vi "Filter(SubVI).vi"(0 "Horní mezní frekvence":dbl, 1 "Vstupní signál":waveform(dbl)[](array[waveform]), 2 "Druh filtru":T1, 3 "Dolní mezní frekvence":dbl, 4 "Vstup z registru":dbl[](array[numeric]), 5 "Typ filtru":bool) -> (6 "Signál":waveform(dbl)[](array[waveform]), 7 "Spektrum":cluster{"f0":dbl, "df":dbl, "magnitude":dbl[]}[](array[cluster]), 8 "Výstup filtrovaného signálu":dbl[](array[numeric]))   [LabVIEW 2025]
doc: "Celkem obsahuje 6 vstupů:\n 1. Vstupní signál pro filtraci\n 2. Horní mezní frekvenci filtru\n 3. Dolní mezní frekvenci filtru (jedinou mezní frekvenci pro filtry DP a HP)\n 4. Přepínač pro typ filtru\n 5. Výběr druhu filtru (HP, DP, PP, PZ)\n 6. Vstup pro kontrolu signálu\nObsahuje 3 výstupy:\n 1. Výstupní vyfiltrovaný signál + původní nefiltrovaný signál\n 2. Spektra obou signálů\n 3. Výstup filtrovaného signálu pro kontrolu\n\nV závislosti na pozici boolean tlačítka se využívá buď FIR filtr, pokud je tlačítko ve stavu OFF, nebo IIR filtr, pokud je tlačítko ve stavu ON."
uses:
  <vilib>/Analysis/NI_AALBase.lvlib
  <vilib>/measure/NI_MAPro.lvlib
  <vilib>/measure/maspectr.llb/FFT Spectrum (Mag-Phase) for N Chan.vi
  <vilib>/Analysis/3filter.llb/Butterworth Filter (DBL).vi
  <vilib>/Analysis/3filter.llb/FIR Filter (DBL).vi
  <vilib>/Analysis/3filter.llb/Filter Passband Type.ctl
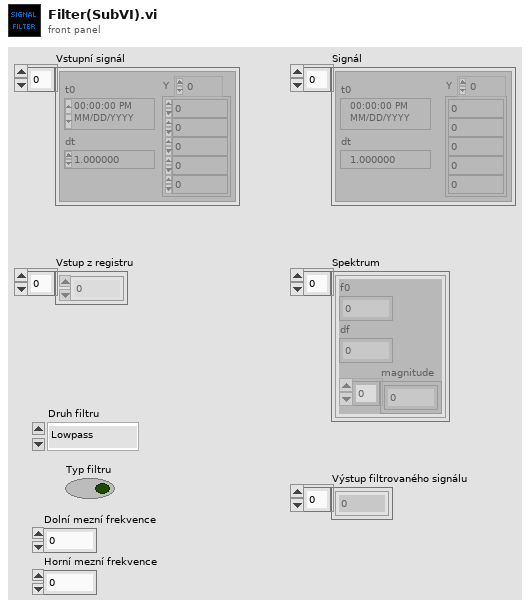
[diagram p1: front panel]
types:
  T1 = typedef "NI_AALBase.lvlib/Filter Passband Type.ctl" = enum32{"Lowpass", "Highpass", "Bandpass", "Bandstop"}
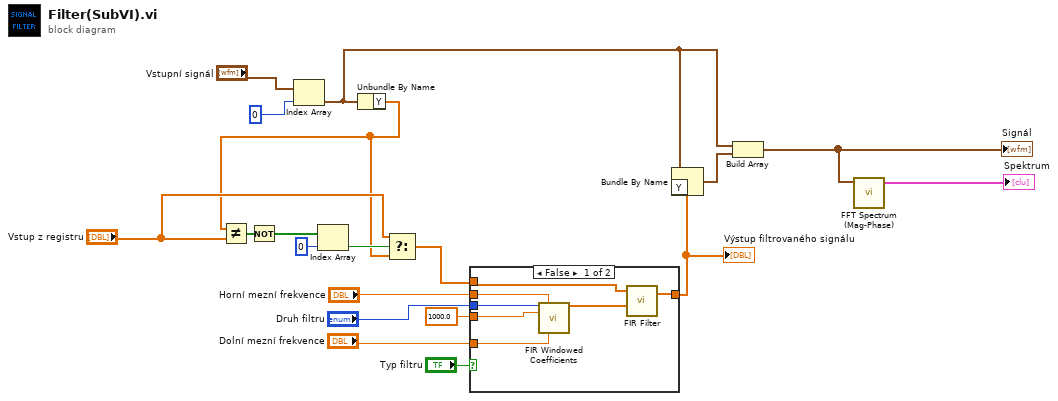
[diagram p0: block diagram]
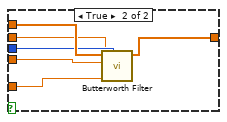
[diagram p2: hidden frame]
diagram:
  n1 = Index Array(array="Vstupní signál", index=0) -> (element=w19:waveform(dbl))
  n2 = Unbundle By Name(w19) -> ("Y"=w5:dbl[])
  n3 = Not Equal?(x=w5, y="Vstup z registru") -> (x != y?=w13:bool[])
  n4 = Not(x=w13) -> (.not. x?=w14:bool[])
  n5 = Index Array(array=w14, index=0) -> (element=w12:bool)
  n6 = Select(t="Vstup z registru", s=w12, f=w5) -> (s? t:f=w16:dbl[])
  n7 = case shown="False" "Typ filtru" {
    tunnel: w16 -> [w25 w32]
    tunnel: "Druh filtru" -> [w20 w31]
    tunnel: 1000.0 ("dt") -> [w22 w30]
    tunnel: "Horní mezní frekvence" -> [w21 w29]
    tunnel: "Dolní mezní frekvence" -> [w23 w28]
    tunnel: [w24 w27] -> w15
    frame False {
      n8 = call <vilib>:"FIR Windowed Coefficients.vi"("filter type"=w20, "high cutoff freq: fh"=w21, "sampling freq: fs"=w22, "low cutoff freq: fl"=w23) -> ("FIR Windowed Coefficients"=w26:dbl[])  [unwired: 10 in, 1 out]
      n9 = call-poly <vilib>:"FIR Filter.vi"("FIR Coefficients"=w26, "X"=w25) -> ("Filtered X"=w24:dbl[])  [unwired: 2 in, 1 out]
    }
    frame True {
      n10 = call-poly <vilib>:"Butterworth Filter.vi"("filter type"=w31, "low cutoff freq: fl"=w28, "high cutoff freq: fh"=w29, "sampling freq: fs"=w30, "X"=w32) -> ("Filtered X"=w27:dbl[])  [unwired: 3 in, 1 out]
    }
  }
  "Výstup filtrovaného signálu" <- w15
  n11 = Bundle By Name ("Build Waveform")(cluster=w19, "Y"=w15) -> (w17:waveform(dbl))
  n12 = Build Array(w19, w17) -> (w18:waveform(dbl)[])
  "Signál" <- w18
  n13 = call-poly <vilib>:"FFT Spectrum (Mag-Phase).vi"("time signals"=w18) -> ("magnitudes"=→"Spektrum":cluster{"f0":dbl, "df":dbl, "magnitude":dbl[]}[])  [unwired: 6 in, 4 out]
